vi "Pose_AlmostEquals.vi"(6 "Tolerance":dbl=1e-05 format="%#_13g", 9 "other POSE":T1 {"ROTATION"."SIN" format="%13.4f"; "ROTATION"."COS" format="%13.4f"; "ROTATION"."VALUE" format="%13.4f"; "TRANSLATION"."Y" format="%14.3f"; "TRANSLATION"."X" format="%14.3f"}, 11 "in POSE":T1 {"ROTATION"."SIN" format="%13.4f"; "ROTATION"."COS" format="%13.4f"; "ROTATION"."VALUE" format="%13.4f"; "TRANSLATION"."Y" format="%14.3f"; "TRANSLATION"."X" format="%14.3f"}) -> (3 "Equals":bool)   [LabVIEW 2019]
doc: "Checks equality between this Pose2d and another Pose2d.\n\nParameters:\n - this Pose - This POSE2D data structure\n - other POSE - The other POSE2d data structure\n\nReturns: \n - Equals - Value will be TRUE if both POSEs are the same"
uses:
  <vilib>/Rock Robotics/WPI/ThirdParty/JAS_Junk/TrajLib/POSE2D.ctl
  <vilib>/Rock Robotics/WPI/ThirdParty/JAS_Junk/TrajLib/TRANSLATION2D.ctl
  <vilib>/Rock Robotics/WPI/ThirdParty/JAS_Junk/TrajLib/ROTATION2D.ctl
  <vilib>/Rock Robotics/WPI/ThirdParty/JAS_Junk/TrajLib/Util_CalcDist.vi
  <vilib>/Rock Robotics/WPI/ThirdParty/JAS_Junk/TrajLib/Trajectory_Library.lvlib
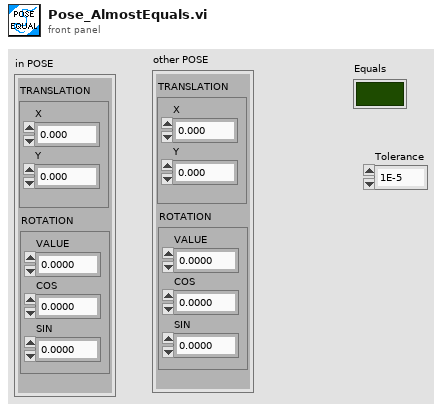
[diagram p1: front panel]
types:
  T1 = typedef "Trajectory_Library.lvlib/POSE2D.ctl" = cluster{"TRANSLATION":T2, "ROTATION":T3}
  T2 = typedef "Trajectory_Library.lvlib/TRANSLATION2D.ctl" = cluster{"X":dbl, "Y":dbl}
  T3 = typedef "Trajectory_Library.lvlib/ROTATION2D.ctl" = cluster{"VALUE":dbl, "COS":dbl, "SIN":dbl}
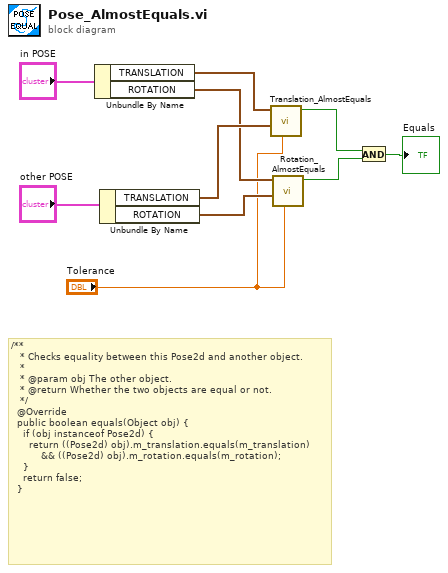
[diagram p0: block diagram]
diagram:
  # "/**\n   * Checks equality between this Pose2d and another object.\n   *\n   * @param obj The other object.\n   * @return Whether the two objects are equal or not.\n   */\n  @Override\n  public boolean equals(Object obj) {\n    if (obj instanceof Pose2d) {\n      return ((Pose2d) obj).m_translation.equals(m_translation)\n          && ((Pose2d) obj).m_rotation.equals(m_rotation);\n    }\n    return false;\n  }"
  n1 = Unbundle By Name("in POSE") -> ("TRANSLATION"=w7:T2, "ROTATION"=w5:T3)
  n2 = Unbundle By Name("other POSE") -> ("TRANSLATION"=w6:T2, "ROTATION"=w4:T3)
  n3 = call "Translation_AlmostEquals.vi"("Tolerance"="Tolerance", "other Translation"=w6, "In Translation"=w7) -> ("Equals"=w3:bool)  [unwired: 8 in]
  n4 = call "Rotation_AlmostEquals.vi"("Tolerance"="Tolerance", "other ROTATION"=w4, "in ROTATION"=w5) -> ("Equals"=w2:bool)  [unwired: 8 in]
  n5 = And(x=w3, y=w2) -> (x .and. y?=→"Equals":bool)
